vi "File Dir Exists.vi"(8 "error in (no error)":errorcluster, 11 "path":path) -> (0 "error out":errorcluster, 2 "exists":bool, 3 "path out":path)   [LabVIEW 2014, in "lvprj2html.lvlib"]
uses:
  lvprj2html.lvlib
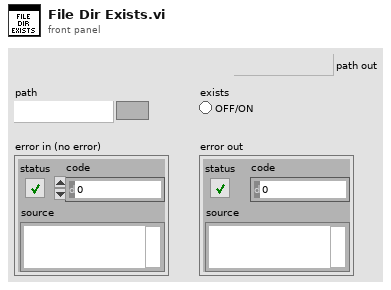
[diagram p1: front panel]
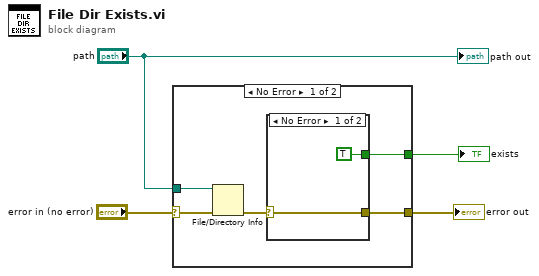
[diagram p0: block diagram]
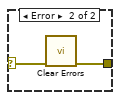
[diagram p2: hidden frame]
diagram:
  n1 = case shown="No Error" "error in (no error)" {
    selector: "error in (no error)" -> [w8 w14]
    tunnel: "path" -> [w9 _]
    tunnel: [w6 w14] -> w3
    tunnel: [w5 _] -> w4
    frame No Error {
      n2 = File/Directory Info(path=w9, error in=w8) -> (error out=w7:errorcluster)  [unwired: 6 out]
      n3 = case shown="No Error" w7 {
        selector: w7 -> [w11 w13]
        tunnel: [w11 w12] -> w6
        tunnel: [TRUE _] -> w5
        frame No Error {
        }
        frame Error {
          n4 = call <vilib>:"Clear Errors.vi"("error in (no error)"=w13) -> ("error out"=w12:errorcluster)  [unwired: 5 in, 1 out]
        }
      }
    }
    frame Error {
    }
  }
  "exists" <- w4
  "error out" <- w3
  "path out" <- "path"
